vi "运维调试_综合生物毒性.vi"() -> ()   [LabVIEW 2016, in "综合生物毒性.lvlib"]
uses:
  <vilib>/Utility/miscctls.llb/LVPointTypeDef.ctl
  <vilib>/Plasmionique/MB Master/MB_Master_Serial/MB_Master_Serial.lvclass
  C:/Program Files (x86)/National Instruments/LabVIEW 2016/vi.lib/Plasmionique/MB Master/MB_Master/MB_Master.lvclass
  <vilib>/Utility/config.llb/NI_LVConfig.lvlib
  <vilib>/Plasmionique/MB Master/MB Master.lvlib
  <vilib>/ptbypt/NI_PtbyPt.lvlib
panel:
  out "测量模式":string
  out "seconds current":timestamp
  out "seconds record":timestamp
  out "工作中":bool
  out "串口号":string
  out "通讯时长":string
  out "通讯":bool
  in  "参数设置":bool
  out "试剂余量":u32
  out "CF":sgl format="%#.6f"
  in  "综合生物毒性":bool=TRUE
  out "培养仓温度":sgl format="%#.2f ℃"
  out "固件版本号":string
  out "模块版本号":string
  out "质控测量结果":sgl format="%#.2f"
  out "水样测量结果":sgl format="%#.2f "
  out "测量仓温度":sgl format="%#.2f ℃"
  out "St":i32
  out "Rt":i32
  out "S0":i32
  out "R0":i32
  out "运行状态":T1 {"数据时间:" format="%<%y/%m/%d %H:%M:%S>T"; "仪器时间:" format="%<%y/%m/%d %H:%M:%S>T"}
  out "集成报警信息":string
  in  "停止":bool
  in  "启动水样测量":bool
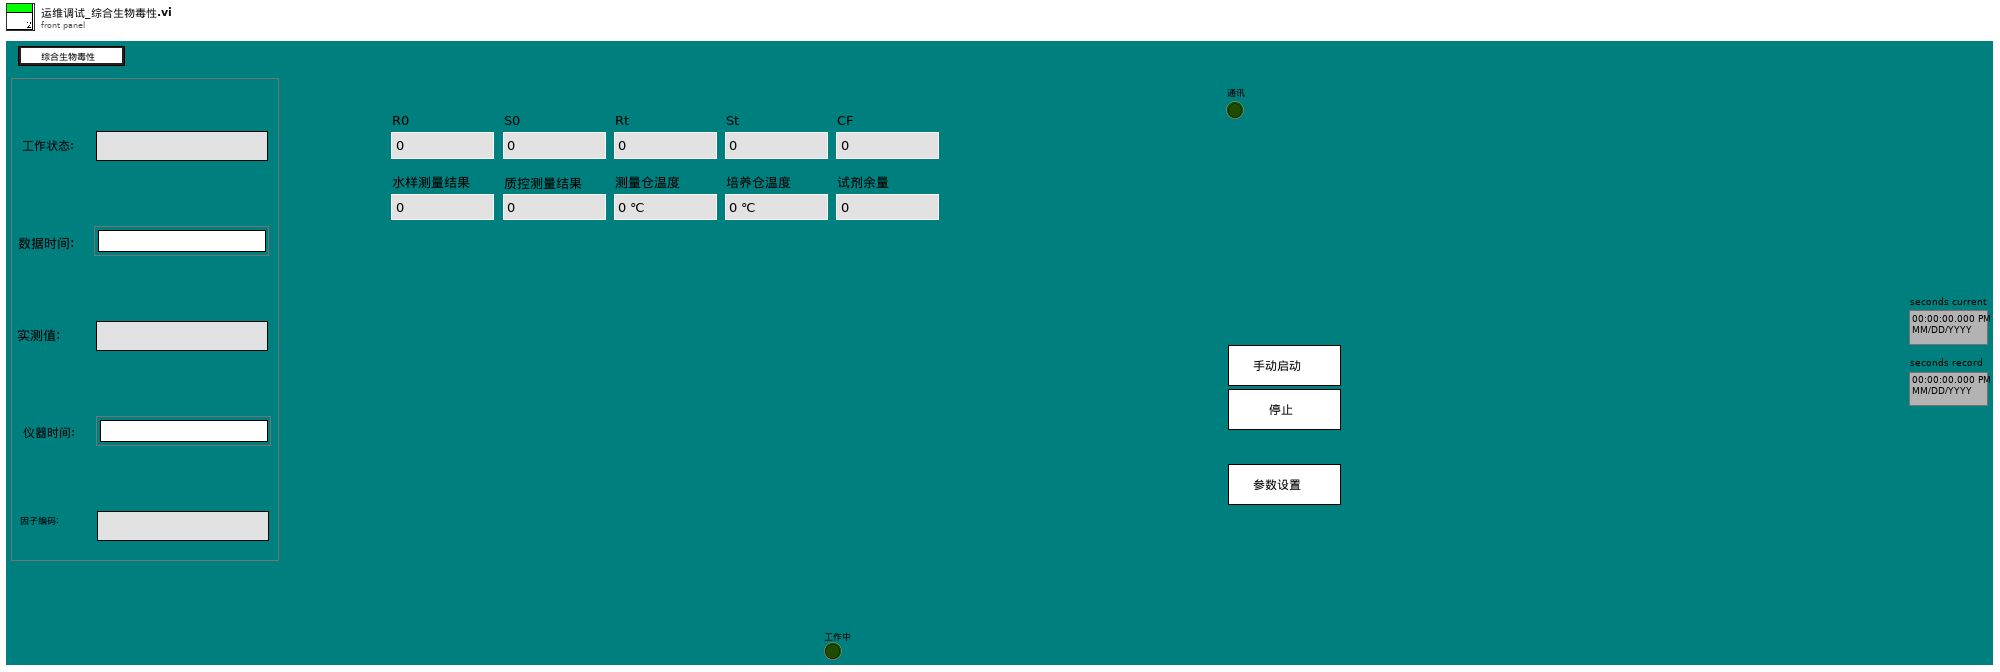
[diagram p1: front panel]
types:
  T1 = cluster{"工作状态:":string, "数据时间:":timestamp, "实测值:":string, "仪器时间:":timestamp, "因子编码:":string}
  T2 = typedef "LVPointTypeDef.ctl" = cluster{"Horizontal":i16, "Vertical":i16}
  T3 = cluster{"Major":u16, "Minor":u16, "Fix":u16, "Build":u16}
  T4 = typedef "NI_LVConfig.lvlib/Config Data RefNum.ctl" = refnum<k1>
  T5 = cluster{"baud rate (bps)":u32, "stop bits":u16, "parity":u16, "flow control":u16, "timeout":u32, "retries":i32}
  T6 = cluster{"时间":timestamp, "水样测量结果":sgl, "质控测量结果":sgl, "R0":i32, "S0":i32, "Rt":i32, "St":i32, "CF":sgl, "测量仓温度":sgl, "培养仓温度":sgl, "试剂余量":u32, "仪器状态":string, "空白结果":dbl, "启动测量":enum32{"无", "启动水样测量", "启动质控测量", "启动纯水测量", "启动自动复苏", "启动自动清洗"}, "停止测量":bool}
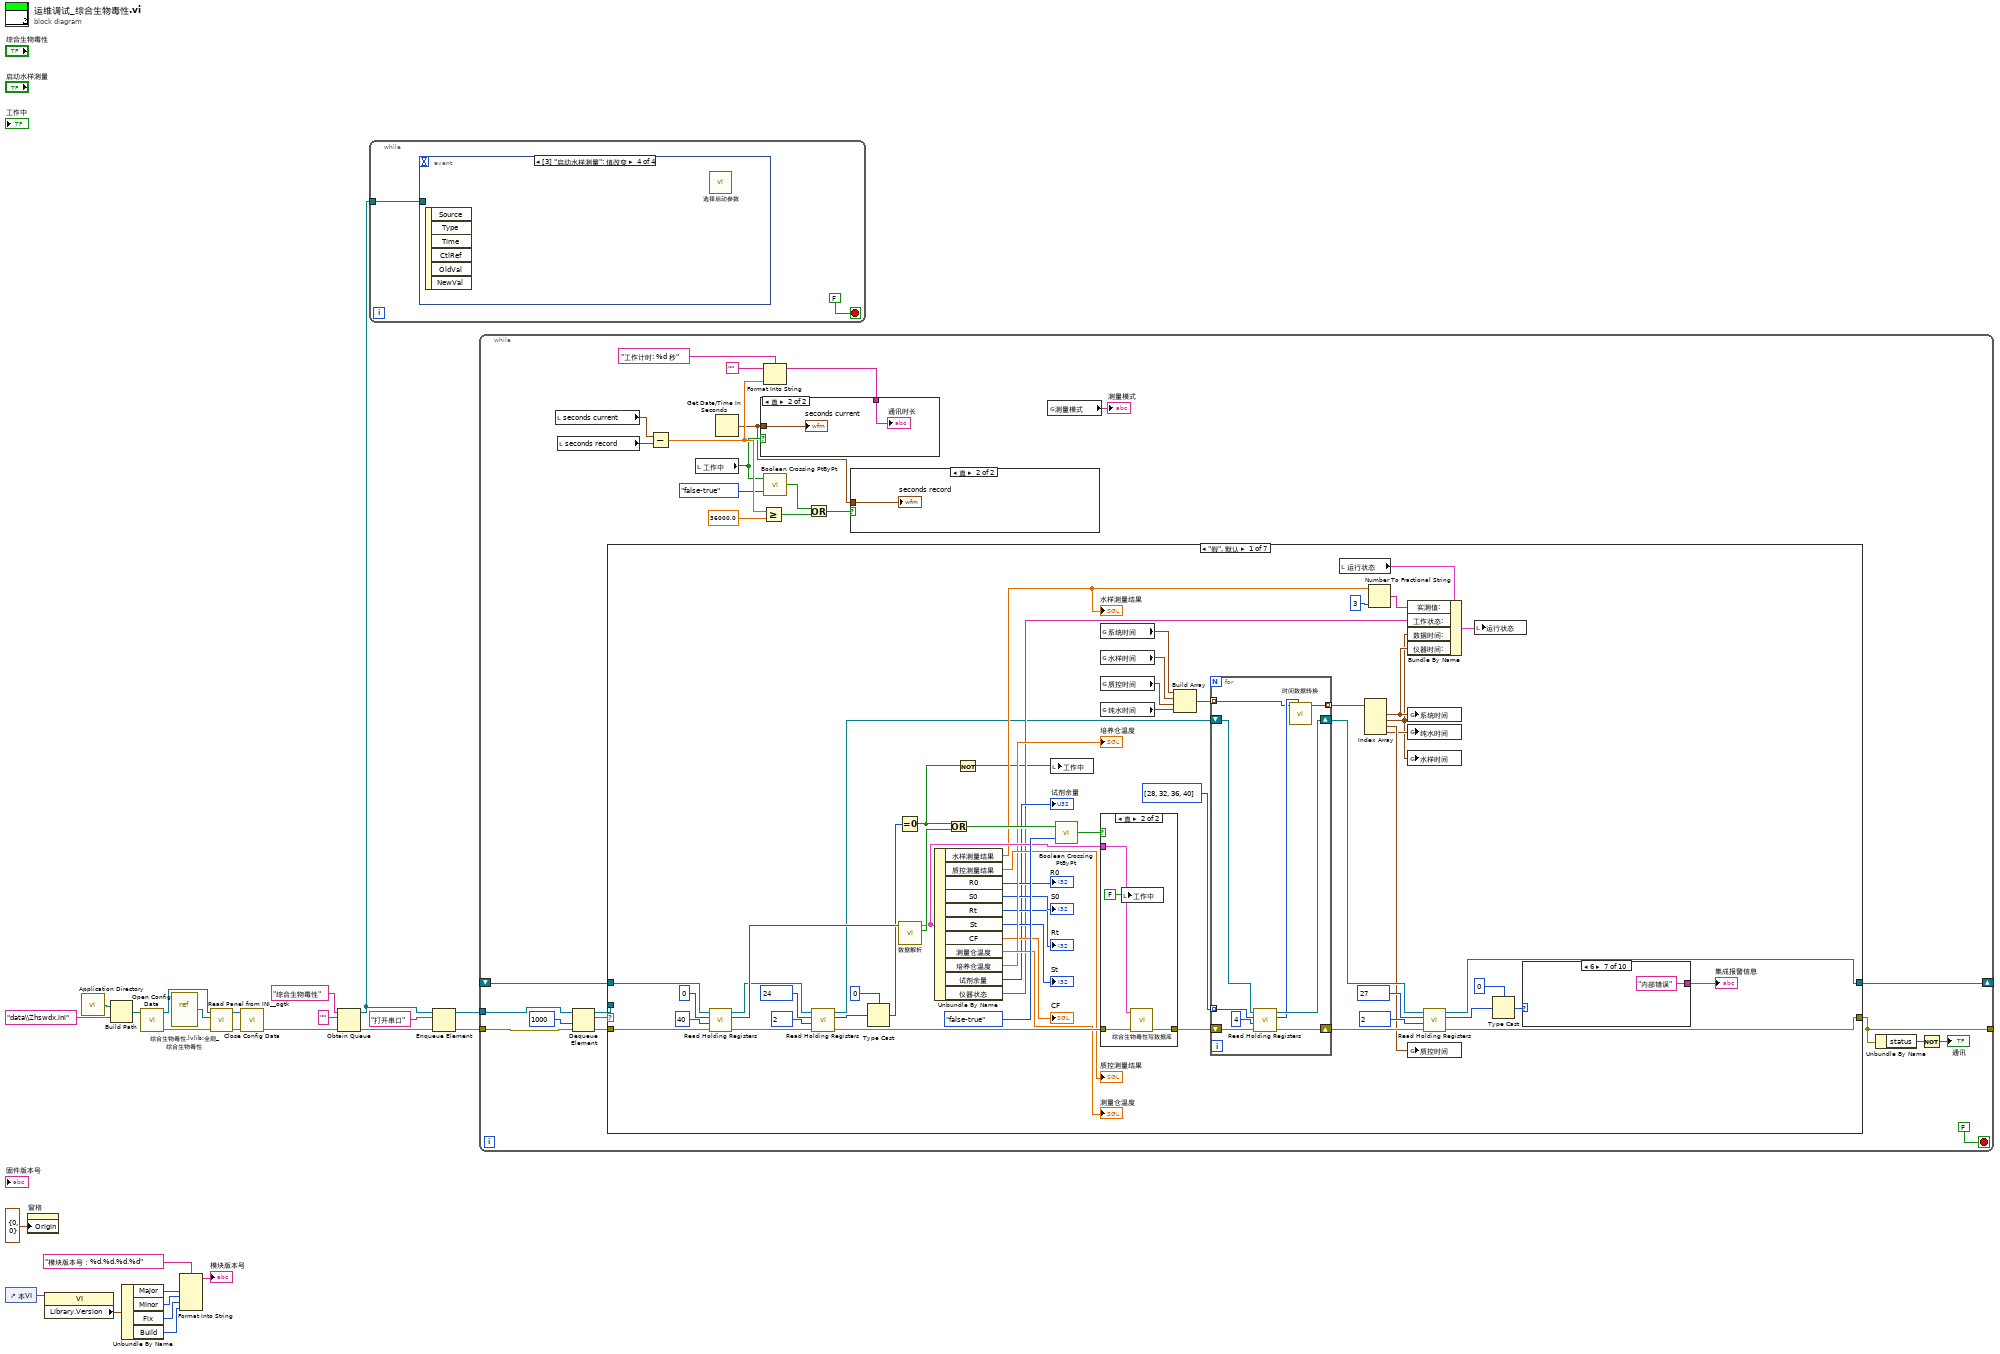
[diagram p0: block diagram]
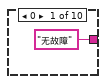
[diagram p4: hidden frame]
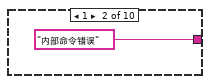
[diagram p5: hidden frame]
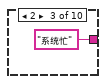
[diagram p6: hidden frame]
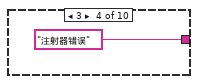
[diagram p7: hidden frame]
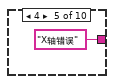
[diagram p8: hidden frame]
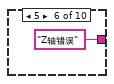
[diagram p9: hidden frame]
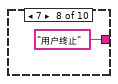
[diagram p10: hidden frame]
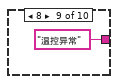
[diagram p11: hidden frame]
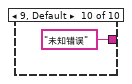
[diagram p12: hidden frame]
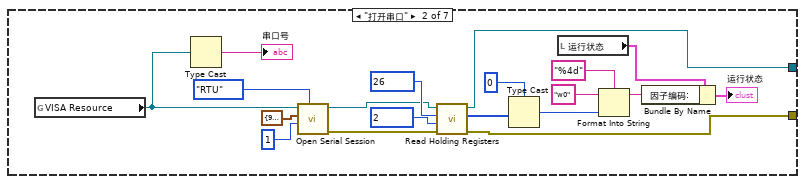
[diagram p14: hidden frame]
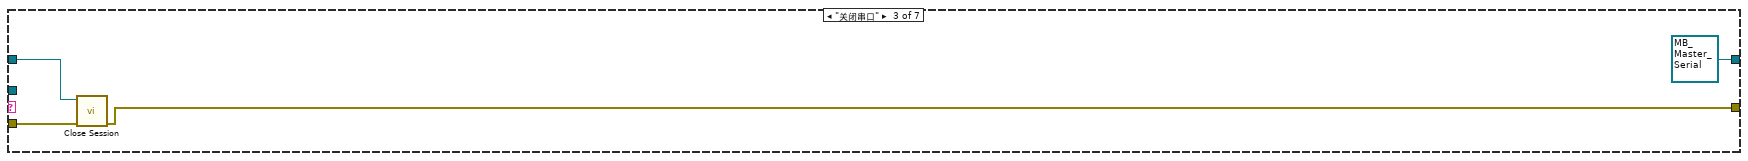
[diagram p15: hidden frame]
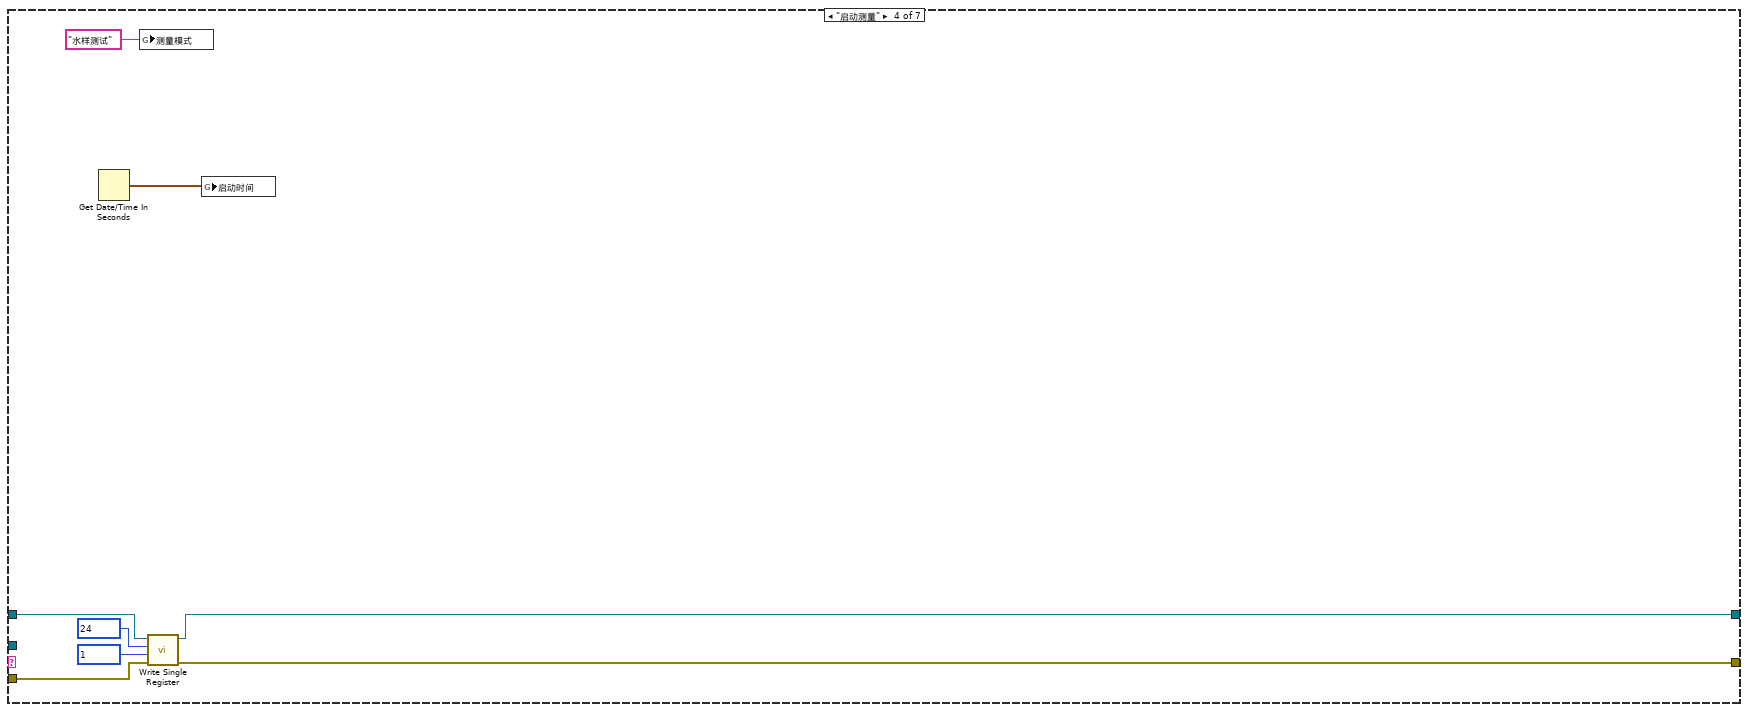
[diagram p16: hidden frame]
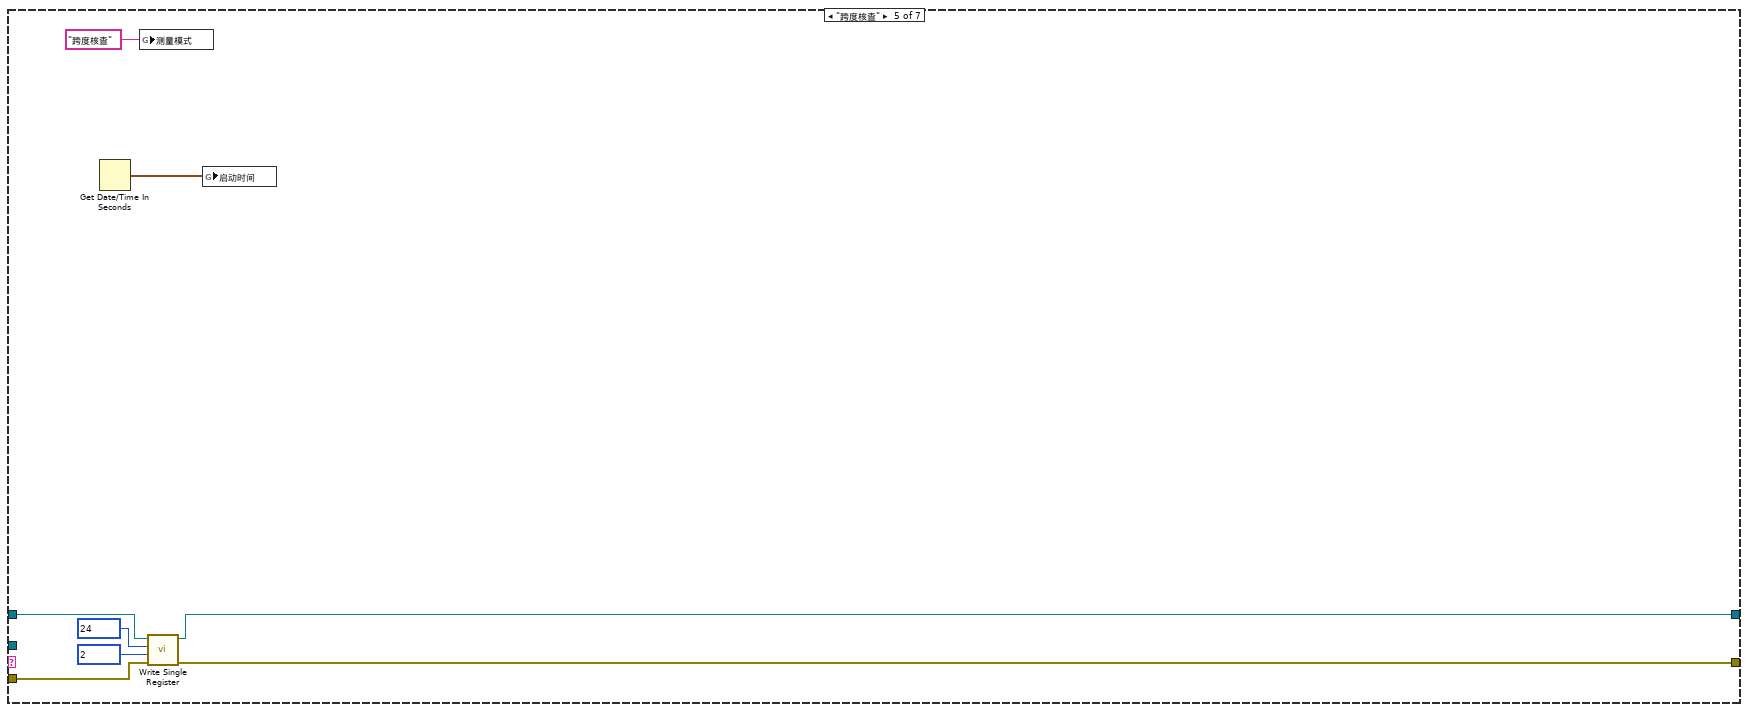
[diagram p17: hidden frame]
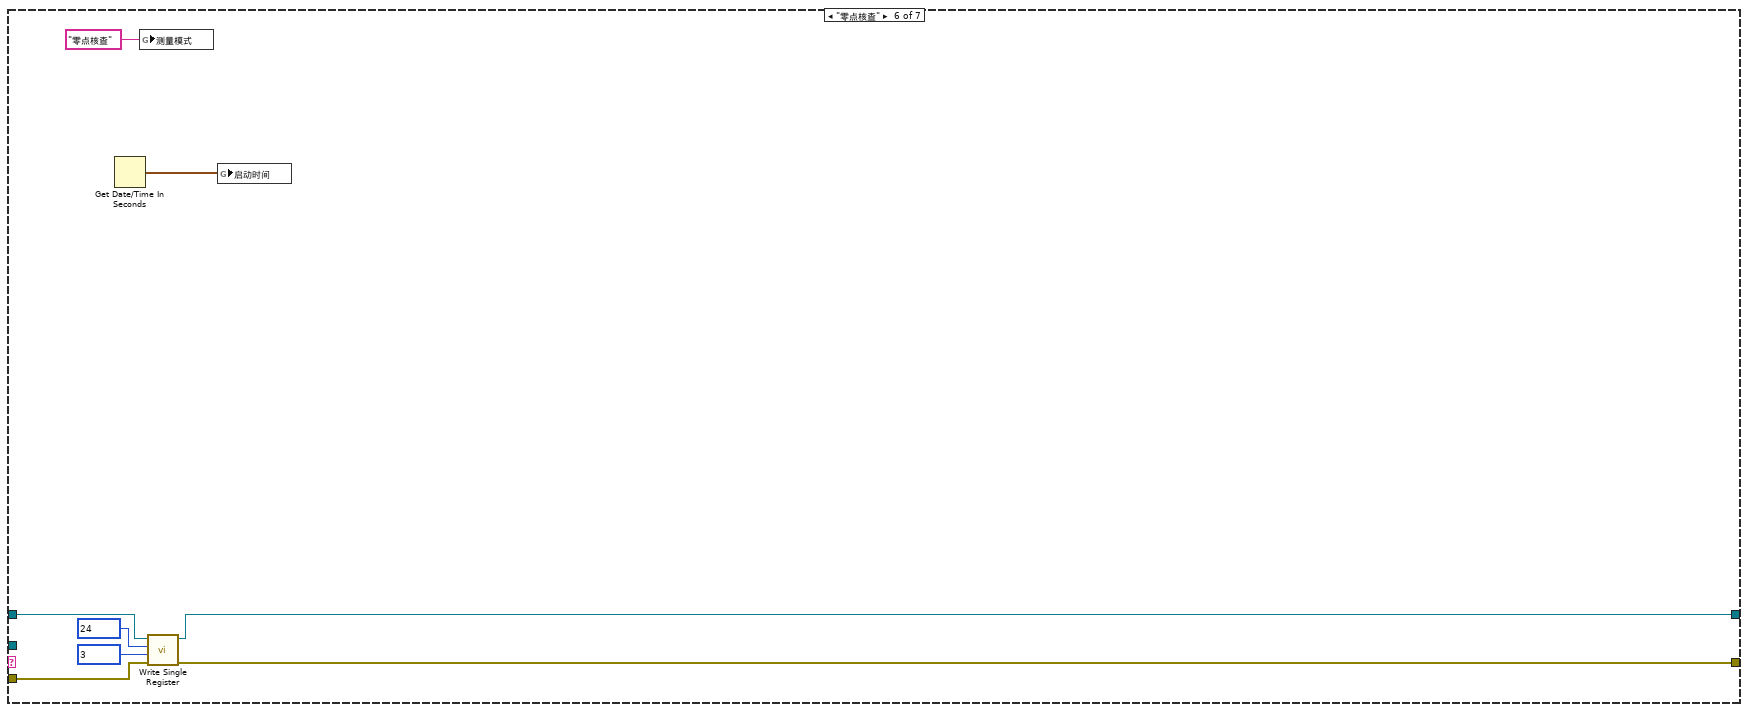
[diagram p18: hidden frame]
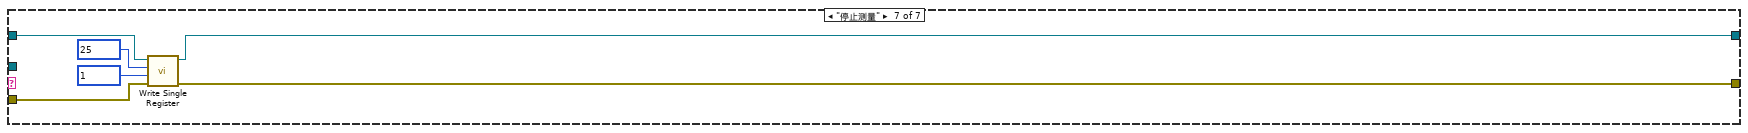
[diagram p19: hidden frame]
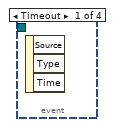
[diagram p20: hidden frame]
diagram:
  n1 = control-ref of="本VI"() -> (w9:refnum<vi>)
  n2 = property on="窗格" class="Pane"("Origin"=T2 {"Horizontal"=0, "Vertical"=0} ("原点")) -> ()  [unwired: 2 in, 2 out]
  n3 = property class="VI"(reference=w9) -> ("Library.Version"=w8:T3)  [unwired: 1 in, 2 out]
  n4 = call <vilib>:"Application Directory.vi"() -> ("Application Directory"=w21:path)
  n5 = Build Path(base path=w21, name or relative path="data\\Zhswdx.ini" ("名称或相对路径")) -> (appended path=w23:path)
  n6 = Unbundle By Name(w8) -> ("Major"=w6:u16, "Minor"=w5:u16, "Fix"=w4:u16, "Build"=w3:u16)
  n7 = call <vilib>:"Open Config Data.vi"("configuration file path"=w23) -> ("error out"=w19:errorcluster, "refnum"=w24:T4)  [unwired: 8 in, 1 out]
  n8 = vi-ref "综合生物毒性.lvlib:全局_综合生物毒性.vi"() -> (w18:refnum<vi>)
  n9 = Format Into String(format string="模块版本号：%d.%d.%d.%d" ("格式字符串"), w6, w5, w4, w3) -> (resulting string=→"模块版本号":string)  [unwired: 2 in, 1 out]
  n10 = call <userlib>:"Read Panel from INI__ogtk.vi"("error in (no error)"=w19, "VI ref"=w18, "refnum"=w24) -> ("error out"=w20:errorcluster, "refnum out"=w25:T4)  [unwired: 7 in]
  n11 = call <vilib>:"Close Config Data.vi"("error in (no error)"=w20, "refnum"=w25) -> ("error out"=w15:errorcluster)  [unwired: 8 in, 1 out]
  n12 = Obtain Queue(name (unnamed)="综合生物毒性" ("名称（未命名）"), element data type="" ("状态"), error in (no error)=w15) -> (queue out=w12:refnum<queue>, error out=w13:errorcluster)  [unwired: 2 in, 1 out]
  n13 = while {
    tunnel: w12 -> [w26]
    stop <- FALSE stop-if-true
    n14 = event shown="[3] \"启动水样测量\": 值改变" {
      selector: _ -> [_ _ _ _]
      dyn-events: _ -> [_ _ _ _]
      timeout: _ -> [_ _ _ _]
      tunnel: w26 -> [_ w28 w37 _]
      event Timeout {
        n15 = event-data() -> ()  [unwired: 1 in, 3 out]
      }
      event "参数设置": Value Change {
        n16 = event-data() -> ()  [unwired: 1 in, 6 out]
        n17 = call "综合生物毒性设置窗口.vi"() -> ("开关"=w29:bool, "确定输出"=w30:bool)  [unwired: 9 in, 1 out]
        n18 = case shown="真" w30 {
          tunnel: w29 -> [_ w35]
          tunnel: w28 -> [_ w31]
          frame False {
          }
          frame True {
            n19 = Select(t="打开串口" ("状态"), s=w35, f="关闭串口" ("状态")) -> (s? t:f=w32:string)
            n20 = Enqueue Element(queue=w31, element=w32) -> ()  [unwired: 2 in, 3 out]
          }
        }
      }
      event "停止": Value Change {
        n21 = event-data() -> ()  [unwired: 1 in, 6 out]
        n22 = Enqueue Element(queue=w37, element="停止测量" ("元素")) -> ()  [unwired: 2 in, 3 out]
      }
      event "启动水样测量": Value Change {
        n23 = event-data() -> ()  [unwired: 1 in, 6 out]
        n24 = call "选择启动参数.vi"() -> ()  [unwired: 12 in]
      }
    }
  }
  n25 = Enqueue Element(queue=w12, element="打开串口" ("状态"), error in (no error)=w13) -> (queue out=w11:refnum<queue>, error out=w10:errorcluster)  [unwired: 1 in, 1 out]
  n26 = while {
    tunnel: w11 -> [w62]
    shift-right: [w56] -> _
    shift-left: _ -> [w55]
    tunnel: w10 -> [w61]
    tunnel: [w41] -> _
    stop <- FALSE stop-if-true
    n27 = local read "seconds current"() -> (w52:timestamp)
    n28 = local read "seconds record"() -> (w53:timestamp)
    n29 = Dequeue Element(queue=w62, timeout in ms (-1)=1000 ("超时毫秒(-1)"), error in (no error)=w61) -> (queue out=w58:refnum<queue>, element=w59:string, error out=w57:errorcluster)  [unwired: 1 out]
    n30 = case shown="\"假\", 默认" w59 {
      tunnel: w58 -> [_ _ _ _ _ _ _]
      tunnel: w57 -> [w121 _ w170 w177 w185 w193 w199]
      tunnel: [w81 w150 refnum<class "MB_Master_Serial.lvclass"> refnum ("MB session out") w174 w182 w190 w196] -> w56
      tunnel: [w80 w149 w169 w175 w183 w191 w197] -> w41
      tunnel: w55 -> [w124 _ w171 w178 w186 w194 w200]
      frame "假", Default {
        n31 = call <vilib>:"Read Holding Registers.vi"("error in (no error)"=w121, "quantity"=u16 40, "starting address"=u16 0, "MB session in"=w124) -> ("error out"=w116:errorcluster, "Registers"=w120:u16[], "MB session out"=w117:refnum<class "MB_Master_Serial.lvclass">)  [unwired: 5 in]
        n32 = call <vilib>:"Read Holding Registers.vi"("error in (no error)"=w116, "quantity"=u16 2 ("starting address"), "starting address"=u16 24, "MB session in"=w117) -> ("error out"=w108:errorcluster, "Registers"=w114:u16[], "MB session out"=w90:refnum<class "MB_Master_Serial.lvclass">)  [unwired: 5 in]
        n33 = Type Cast(type=u32 0 ("数字"), x=w114) -> (*(type *) &x=w113:u32)
        n34 = Equal To 0?(x=w113) -> (x = 0?=w70:bool)
        n35 = call "数据解析.vi"("数组"=w120) -> ("空闲"=w112:bool, "综合生物毒性"=w107:T6)  [unwired: 9 in]
        n36 = Unbundle By Name(w107) -> ("水样测量结果"=w96:sgl, "质控测量结果"=→"质控测量结果":sgl, "R0"=→"R0":i32, "S0"=→"S0":i32, "Rt"=→"Rt":i32, "St"=→"St":i32, "CF"=→"CF":sgl, "测量仓温度"=→"测量仓温度":sgl, "培养仓温度"=→"培养仓温度":sgl, "试剂余量"=→"试剂余量":u32, "仪器状态"=w93:string)
        "水样测量结果" <- w96
        n37 = Or(x=w70, y=w112) -> (x .or. y?=w111:bool)
        n38 = Not(x=w70) -> (.not. x?=w69:bool)
        n39 = local write "工作中"(w69) -> ()
        n40 = call <vilib>:"Boolean Crossing PtByPt.vi"("direction"=enum16{"either", "false-true", "true-false"}."false-true", "input"=w111) -> ("crossing"=w109:bool)  [unwired: 1 in]
        n41 = case shown="真" w109 {
          tunnel: w107 -> [_ w148]
          tunnel: w108 -> [w144 w147]
          tunnel: [w144 w146] -> w91
          frame False {
          }
          frame True {
            n42 = local write "工作中"(FALSE ("工作中")) -> ()
            n43 = call "综合生物毒性写数据库.vi"("错误输入（无错误）"=w147, "综合生物毒性"=w148) -> ("错误输出"=w146:errorcluster)  [unwired: 9 in]
          }
        }
        n44 = global read "全局_综合生物毒性.vi" "系统时间"() -> (w78:timestamp)
        n45 = global read "全局_综合生物毒性.vi" "水样时间"() -> (w77:timestamp)
        n46 = global read "全局_综合生物毒性.vi" "质控时间"() -> (w76:timestamp)
        n47 = global read "全局_综合生物毒性.vi" "纯水时间"() -> (w75:timestamp)
        n48 = Build Array(w78, w77, w76, w75) -> (w74:timestamp[])
        n49 = for {
          shift-right: [w141] -> w82
          shift-left: w91 -> [w140]
          shift-right: [w142] -> w83
          shift-left: w90 -> [w143]
          tunnel: u16[] [28, 32, 36, 40] -> [w138] mode=indexing
          tunnel: [w136] -> w73 mode=indexing
          tunnel: w74 -> [w135] mode=indexing
          n50 = call <vilib>:"Read Holding Registers.vi"("error in (no error)"=w140, "quantity"=u16 4, "starting address"=w138, "MB session in"=w143) -> ("error out"=w141:errorcluster, "Registers"=w137:u16[], "MB session out"=w142:refnum<class "MB_Master_Serial.lvclass">)  [unwired: 5 in]
          n51 = call "时间数据转换.vi"("时间寄存器"=w137, "时间"=w135) -> ("time stamp"=w136:timestamp)  [unwired: 8 in, 1 out]
        }
        n52 = local read "运行状态"() -> (w95:T1)
        n53 = Index Array(array=w73) -> (element #1=w68:timestamp, element #2=w67:timestamp, element #3=w72:timestamp, element #4=w71:timestamp)  [unwired: 4 in]
        n54 = Number To Fractional String(number=w96, precision (6)=i16 3 ("精度(6)")) -> (F-format string=w94:string)  [unwired: 2 in]
        n55 = Bundle By Name(cluster=w95, "实测值:"=w94, "工作状态:"=w93, "数据时间:"=w67, "仪器时间:"=w68) -> (w92:T1)
        n56 = global write "全局_综合生物毒性.vi" "系统时间"(w68) -> ()
        n57 = global write "全局_综合生物毒性.vi" "纯水时间"(w71) -> ()
        n58 = global write "全局_综合生物毒性.vi" "水样时间"(w67) -> ()
        n59 = global write "全局_综合生物毒性.vi" "质控时间"(w72) -> ()
        n60 = call <vilib>:"Read Holding Registers.vi"("error in (no error)"=w82, "quantity"=u16 2 ("starting address"), "starting address"=u16 27, "MB session in"=w83) -> ("error out"=w80:errorcluster, "Registers"=w86:u16[], "MB session out"=w81:refnum<class "MB_Master_Serial.lvclass">)  [unwired: 5 in]
        n61 = local write "运行状态"(w92) -> ()
        n62 = Type Cast(type=0, x=w86) -> (*(type *) &x=w88:i32)
        n63 = case shown="6" w88 {
          tunnel: ["无故障" "内部命令错误" "系统忙" "注射器错误" "X轴错误" "Z轴错误" "内部错误" "用户终止" "温控异常" "未知错误"] -> w79
          frame 0 {
          }
          frame 1 {
          }
          frame 2 {
          }
          frame 3 {
          }
          frame 4 {
          }
          frame 5 {
          }
          frame 6 {
          }
          frame 7 {
          }
          frame 8 {
          }
          frame 9, Default {
          }
        }
        "集成报警信息" <- w79
      }
      frame "打开串口" {
        n64 = global read "全局_综合生物毒性.vi" "VISA Resource"() -> (w164:refnum<visa-resource-name>)
        n65 = Type Cast(x=w164) -> (*(type *) &x=→"串口号":string)  [unwired: 1 in]
        n66 = call <vilib>:"Open Serial Session.vi"("Mode (RTU)"=enum16{"RTU", "ASCII"}."RTU", "Slave ID"=u8 1, "Serial Config"=T5 {"baud rate (bps)"=9600, "stop bits"=10, "parity"=0, "flow control"=0, "timeout"=2000, "retries"=1}, "VISA Resource"=w164) -> ("Error out"=w161:errorcluster, "MB_Serial session"=w160:refnum<class "MB_Master_Serial.lvclass">)  [unwired: 6 in]
        n67 = call <vilib>:"Read Holding Registers.vi"("error in (no error)"=w161, "quantity"=u16 2 ("starting address"), "starting address"=u16 26, "MB session in"=w160) -> ("error out"=w149:errorcluster, "Registers"=w158:u16[], "MB session out"=w150:refnum<class "MB_Master_Serial.lvclass">)  [unwired: 5 in]
        n68 = Type Cast(type=0, x=w158) -> (*(type *) &x=w155:i32)
        n69 = local read "运行状态"() -> (w152:T1)
        n70 = Format Into String(format string="%4d" ("格式字符串"), initial string="w0" ("初始字符串"), w155) -> (resulting string=w154:string)  [unwired: 1 in, 1 out]
        n71 = Bundle By Name(cluster=w152, "因子编码:"=w154) -> (→"运行状态":T1)
      }
      frame "关闭串口" {
        n72 = call-dynamic "Close Session.vi"("error in (no error)"=w170, "MB_Serial session"=w171) -> ("error out"=w169:errorcluster)  [unwired: 9 in]
      }
      frame "启动测量" {
        n73 = Get Date/Time In Seconds() -> (seconds since 1Jan1904=w172:timestamp)
        n74 = global write "全局_综合生物毒性.vi" "测量模式"("水样测试" ("运行模式")) -> ()
        n75 = call <vilib>:"Write Single Register.vi"("error in (no error)"=w177, "value"=u16 1 ("starting address"), "address"=u16 24 ("starting address"), "MB session in"=w178) -> ("error out"=w175:errorcluster, "MB session out"=w174:refnum<class "MB_Master_Serial.lvclass">)  [unwired: 6 in]
        n76 = global write "全局_综合生物毒性.vi" "启动时间"(w172) -> ()
      }
      frame "跨度核查" {
        n77 = Get Date/Time In Seconds() -> (seconds since 1Jan1904=w180:timestamp)
        n78 = global write "全局_综合生物毒性.vi" "测量模式"("跨度核查" ("运行模式")) -> ()
        n79 = call <vilib>:"Write Single Register.vi"("error in (no error)"=w185, "value"=u16 2 ("starting address"), "address"=u16 24 ("starting address"), "MB session in"=w186) -> ("error out"=w183:errorcluster, "MB session out"=w182:refnum<class "MB_Master_Serial.lvclass">)  [unwired: 6 in]
        n80 = global write "全局_综合生物毒性.vi" "启动时间"(w180) -> ()
      }
      frame "零点核查" {
        n81 = Get Date/Time In Seconds() -> (seconds since 1Jan1904=w188:timestamp)
        n82 = global write "全局_综合生物毒性.vi" "测量模式"("零点核查" ("运行模式")) -> ()
        n83 = call <vilib>:"Write Single Register.vi"("error in (no error)"=w193, "value"=u16 3 ("starting address"), "address"=u16 24 ("starting address"), "MB session in"=w194) -> ("error out"=w191:errorcluster, "MB session out"=w190:refnum<class "MB_Master_Serial.lvclass">)  [unwired: 6 in]
        n84 = global write "全局_综合生物毒性.vi" "启动时间"(w188) -> ()
      }
      frame "停止测量" {
        n85 = call <vilib>:"Write Single Register.vi"("error in (no error)"=w199, "value"=u16 1 ("starting address"), "address"=u16 25 ("starting address"), "MB session in"=w200) -> ("error out"=w197:errorcluster, "MB session out"=w196:refnum<class "MB_Master_Serial.lvclass">)  [unwired: 6 in]
      }
    }
    n86 = Subtract(x=w52, y=w53) -> (x-y=w54:dbl)
    n87 = local read "工作中"() -> (w49:bool)
    n88 = Get Date/Time In Seconds() -> (seconds since 1Jan1904=w44:timestamp)
    n89 = Greater Or Equal?(x=w54, y=36000.0) -> (x >= y?=w47:bool)
    n90 = Format Into String(format string="工作计时: %d 秒" ("格式字符串"), initial string="", w54) -> (resulting string=w39:string)  [unwired: 1 in, 1 out]
    n91 = case shown="真" w49 {
      tunnel: w44 -> [_ w65]
      tunnel: w39 -> [_ w64]
      frame False {
      }
      frame True {
        "seconds current" <- w65
        "通讯时长" <- w64
      }
    }
    n92 = call <vilib>:"Boolean Crossing PtByPt.vi"("direction"=enum16{"either", "false-true", "true-false"}."false-true", "input"=w49) -> ("crossing"=w46:bool)  [unwired: 1 in]
    n93 = Or(x=w46, y=w47) -> (x .or. y?=w48:bool)
    n94 = case shown="真" w48 {
      tunnel: w44 -> [_ w66]
      frame False {
      }
      frame True {
        "seconds record" <- w66
      }
    }
    n95 = global read "全局_综合生物毒性.vi" "测量模式"() -> (→"测量模式":string)
    n96 = Unbundle By Name(w41) -> ("status"=w42:bool)
    n97 = Not(x=w42) -> (.not. x?=→"通讯":bool)
  }
